vi "UnLoad.vi"(8 "error in (no error)":errorcluster) -> (0 "error out":errorcluster)   [LabVIEW 2020, in "WebServiceImporter.lvlib" / "Main Panel.lvlib" / "Input Info.lvlib"]
uses:
  <vilib>/Platform/WebService/Main Panel/Pages/Input Info/Input Info.lvlib
  <vilib>/Platform/WebService/Main Panel/Pages/Input Info/Events/Events.lvlib
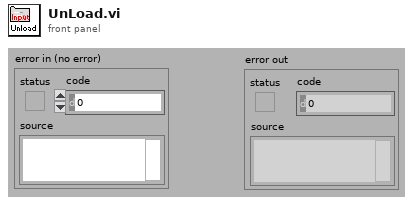
[diagram p1: front panel]
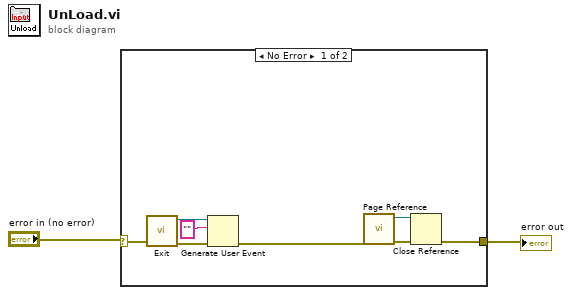
[diagram p0: block diagram]
diagram:
  n1 = case shown="No Error" "error in (no error)" {
    selector: "error in (no error)" -> [w5 w11]
    tunnel: [w9 w11] -> w1
    frame No Error {
      n2 = call <vilib>:"Exit.vi"("error in (no error)"=w5) -> ("error out"=w4:errorcluster, "user event (out)"=w7:refnum<user-event>)  [unwired: 9 in]
      n3 = Generate User Event(user event=w7, event data cluster="" ("event data"), error in=w4) -> (error out=w3:errorcluster)  [unwired: 1 in, 1 out]
      n4 = call <vilib>:"Page Reference.vi"("error in (no error)"=w3) -> ("error out"=w8:errorcluster, "VI Refnum (out)"=w10:refnum<vi>)  [unwired: 9 in]
      n5 = Close Reference(reference=w10, error in (no error)=w8) -> (error out=w9:errorcluster)
    }
    frame Error {
    }
  }
  "error out" <- w1
